vi "test LTS stage.vi"() -> ()   [LabVIEW 2018]
uses:
  Hardware Mfg/Thorlabs Translation Stages/Controls/Motion Translation Module Control.ctl
  Hardware Mfg/Thorlabs Translation Stages/Controls/Translation Stage Cluster.ctl
  General/Controls/Translation Stage Types.ctl
  General/Controls/Set Get Controls.ctl
  C:/Project/SerialSectionOCT/SerialSectOCT/Labview Software/Thorlabs.MotionControl.Controls.dll
  Thorlabs.MotionControl.Controls.dll
panel:
  in  "LTS Reference 2":refnum<k24>(container)
  in  "Set/Get 4":T1=enum."Get"
  in  "Action 4":T2=enum."Stop"
  in  "Set/Get 3":T1=enum."Get"
  in  "Action 3":T2=enum."Stop"
  in  "Set/Get 2":T1=enum."Get"
  in  "Action 2":T2=enum."Stop"
  in  "Cluster In":T3={"Position"=0.0, "Is.Enabled?"=FALSE, "Is.Connected?"=FALSE, "Device SN"="45995820", "AccelerationMaximum"=0.0, "VelocityMaximum"=0.0, "Acceleration"=0.0, "Velocity"=0.0, "waitTimeout (ms)"=10000, "Model"=enum."None", "Is.Homed?"=FALSE}
  in  "Set/Get":T1=enum."Get"
  out "Cluster Out":T3={"Position"=0.0, "Is.Enabled?"=FALSE, "Is.Connected?"=FALSE, "Device SN"="45876539", "AccelerationMaximum"=0.0, "VelocityMaximum"=0.0, "Acceleration"=0.0, "Velocity"=0.0, "waitTimeout (ms)"=0, "Model"=enum."None", "Is.Homed?"=FALSE}
  out "Error Out":errorcluster
  in  "Error In":errorcluster
  in  "Action":T2=enum."Stop"
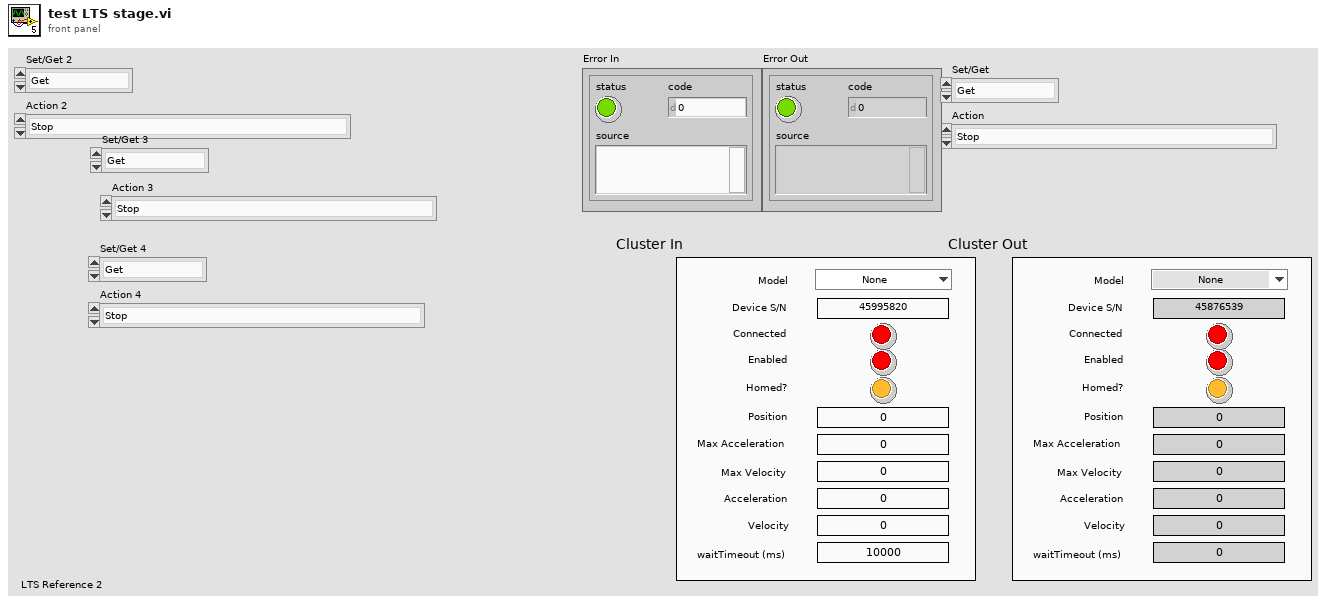
[diagram p1: front panel]
types:
  T1 = typedef "Set Get Controls.ctl" = enum16{"Set", "Get"}
  T2 = typedef "Motion Translation Module Control.ctl" = enum16{"Init", "Home", "Status", "Velocity/Accel", "Position", "Jog", "Stop", "Uninit", "Enable", "Disable"}
  T3 = typedef "Translation Stage Cluster.ctl" = cluster{"Position":dbl, "Is.Enabled?":bool, "Is.Connected?":bool, "Device SN":string, "AccelerationMaximum":dbl, "VelocityMaximum":dbl, "Acceleration":dbl, "Velocity":dbl, "waitTimeout (ms)":i32, "Model":T4, "Is.Homed?":bool}
  T4 = typedef "Translation Stage Types.ctl" = enum16{"None", "Thorlabs LTS", "Thorlabs MLJ"}
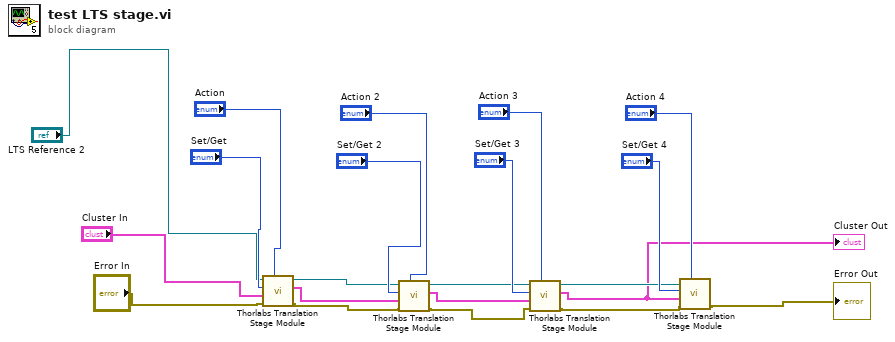
[diagram p0: block diagram]
diagram:
  n1 = call "Thorlabs Translation Stage Module.vi"("Action"="Action", "error in (no error)"="Error In", "Cluster In"="Cluster In", "Set/Get"="Set/Get", ".NET Refnum in"="LTS Reference 2") -> ("error out"=w20:errorcluster, "Cluster out"=w15:T3, ".NET Refnum out"=w5:refnum<k24>)  [unwired: 4 in]
  n2 = call "Thorlabs Translation Stage Module.vi"("Action"="Action 2", "error in (no error)"=w20, "Cluster In"=w15, "Set/Get"="Set/Get 2", ".NET Refnum in"=w5) -> ("error out"=w19:errorcluster, "Cluster out"=w14:T3, ".NET Refnum out"=w4:refnum<k24>)  [unwired: 4 in]
  n3 = call "Thorlabs Translation Stage Module.vi"("Action"="Action 3", "error in (no error)"=w19, "Cluster In"=w14, "Set/Get"="Set/Get 3", ".NET Refnum in"=w4) -> ("error out"=w18:errorcluster, "Cluster out"=w1:T3, ".NET Refnum out"=w3:refnum<k24>)  [unwired: 4 in]
  "Cluster Out" <- w1
  n4 = call "Thorlabs Translation Stage Module.vi"("Action"="Action 4", "error in (no error)"=w18, "Cluster In"=w1, "Set/Get"="Set/Get 4", ".NET Refnum in"=w3) -> ("error out"=→"Error Out":errorcluster)  [unwired: 4 in, 2 out]
